vi "SubVISample.vi"() -> ()   [LabVIEW 2025]
panel:
  in  "action 3":enum16{"", "add\n", "multiply\n", "subtract\n"}(ring)
  in  "action 2":enum16{"", "add\n", "multiply\n", "subtract\n"}(ring)
  in  "action":enum16{"", "add\n", "multiply\n", "subtract\n"}(ring)
  out "result 2":dbl
  out "result 1":dbl
  out "result 3":dbl
  in  "Numeric 8":dbl
  in  "Numeric 7":dbl
  in  "Numeric 6":dbl
  in  "Numeric 5":dbl
  in  "Numeric 4":dbl
  in  "Numeric 3":dbl
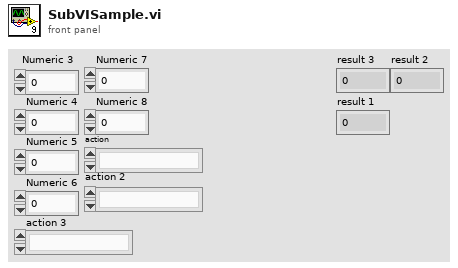
[diagram p1: front panel]
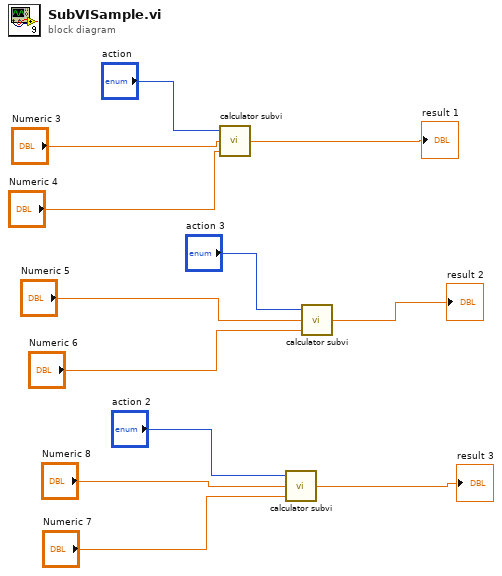
[diagram p0: block diagram]
diagram:
  n1 = call "calculator subvi.vi"("num 5"="Numeric 4", "num 6"="Numeric 3", "Enum"="action") -> ("result"=→"result 1":dbl)
  n2 = call "calculator subvi.vi"("num 5"="Numeric 7", "num 6"="Numeric 8", "Enum"="action 2") -> ("result"=→"result 3":dbl)
  n3 = call "calculator subvi.vi"("num 5"="Numeric 6", "num 6"="Numeric 5", "Enum"="action 3") -> ("result"=→"result 2":dbl)
